vi "Move.vi"(8 "error in (no error)":errorcluster, 10 "Move Data":cluster{"Direction":T1, "Step (px)":u16}, 11 "Geometric Figure in":refnum<class "UI Object.lvclass">) -> (0 "error out":errorcluster, 3 "Geometric Figure out":refnum<class "UI Object.lvclass">)   [LabVIEW 2016, in "PacManClasses.lvlib" / "UI Object.lvclass"]
uses:
  UI Object.lvclass
  Generic Controls/Direction.ctl
  UI Object.lvclass/UI Object.ctl
  Write Center (px).vi
  PacManClasses.lvlib
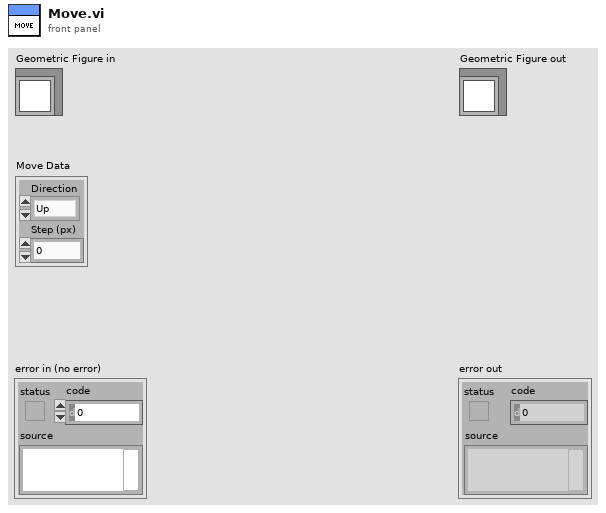
[diagram p1: front panel]
types:
  T1 = typedef "PacManClasses.lvlib/Direction.ctl" = enum16{"Up", "Down", "Left", "Right"}
  T2 = typedef "PacManClasses.lvlib/Point.ctl" = cluster{"x":u16, "y":u16}
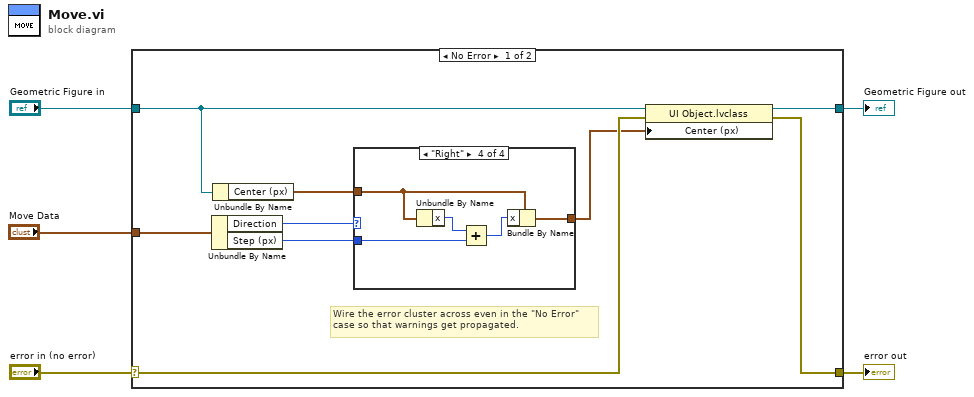
[diagram p0: block diagram]
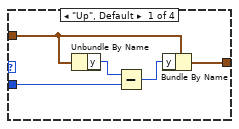
[diagram p2: hidden frame]
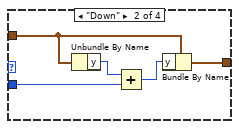
[diagram p3: hidden frame]
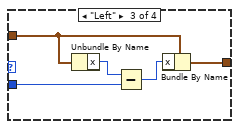
[diagram p4: hidden frame]
diagram:
  n1 = case shown="No Error" "error in (no error)" {
    selector: "error in (no error)" -> [w8 w36]
    tunnel: [w7 w36] -> w4
    tunnel: [w9 w35] -> w2
    tunnel: "Geometric Figure in" -> [w10 w35]
    tunnel: "Move Data" -> [w14 _]
    frame No Error {
      # "Wire the error cluster across even in the \"No Error\"\ncase so that warnings get propagated."
      n2 = Unbundle By Name(w14) -> ("Direction"=w13:T1, "Step (px)"=w11:u16)
      n3 = Unbundle By Name(w10) -> ("Center (px)"=w12:T2)
      n4 = case shown="\"Right\"" w13 {
        tunnel: w12 -> [w19 w24 w29 w34]
        tunnel: w11 -> [w17 w22 w27 w32]
        tunnel: [w15 w20 w25 w30] -> w6
        frame "Up", Default {
          n5 = Unbundle By Name(w19) -> ("y"=w18:u16)
          n6 = Subtract(x=w18, y=w17) -> (x-y=w16:u16)
          n7 = Bundle By Name(cluster=w19, "y"=w16) -> (w15:T2)
        }
        frame "Down" {
          n8 = Unbundle By Name(w24) -> ("y"=w23:u16)
          n9 = Add(x=w23, y=w22) -> (x+y=w21:u16)
          n10 = Bundle By Name(cluster=w24, "y"=w21) -> (w20:T2)
        }
        frame "Left" {
          n11 = Unbundle By Name(w29) -> ("x"=w28:u16)
          n12 = Subtract(x=w28, y=w27) -> (x-y=w26:u16)
          n13 = Bundle By Name(cluster=w29, "x"=w26) -> (w25:T2)
        }
        frame "Right" {
          n14 = Unbundle By Name(w34) -> ("x"=w33:u16)
          n15 = Add(x=w33, y=w32) -> (x+y=w31:u16)
          n16 = Bundle By Name(cluster=w34, "x"=w31) -> (w30:T2)
        }
      }
      n17 = property class="UI Object.lvclass"(reference=w10, error in=w8, "Center (px)"=w6) -> (reference out=w9:refnum<class "UI Object.lvclass">, error out=w7:errorcluster)
    }
    frame Error {
    }
  }
  "error out" <- w4
  "Geometric Figure out" <- w2
